vi "Obtain Message Queue (poly).vi"   [LabVIEW 2018, in "Message Queue.lvlib"]
uses:
  Message Queue.lvlib
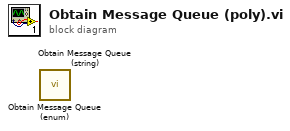
[diagram p0: block diagram]
diagram:
  n1 = call "Obtain Message Queue (enum).vi"() -> ()  [unwired: 10 in, 2 out]
  n2 = call "Obtain Message Queue (string).vi"() -> ()  [unwired: 10 in, 2 out]
